vi "NI 9263 DOUBLE TASK.vi"(8 "error in":errorcluster, 10 "MODULE NAME 2":string="CDR_AO2", 11 "MODULE NAME":string="CDR_AO1") -> (0 "error out":errorcluster, 3 "task out":refnum<k21>)   [LabVIEW 2019]
uses:
  <vilib>/DAQmx/create/channels.llb/DAQmx Create Channel (AO-Voltage-Basic).vi
  <resource>/objmgr/daqmx.rc
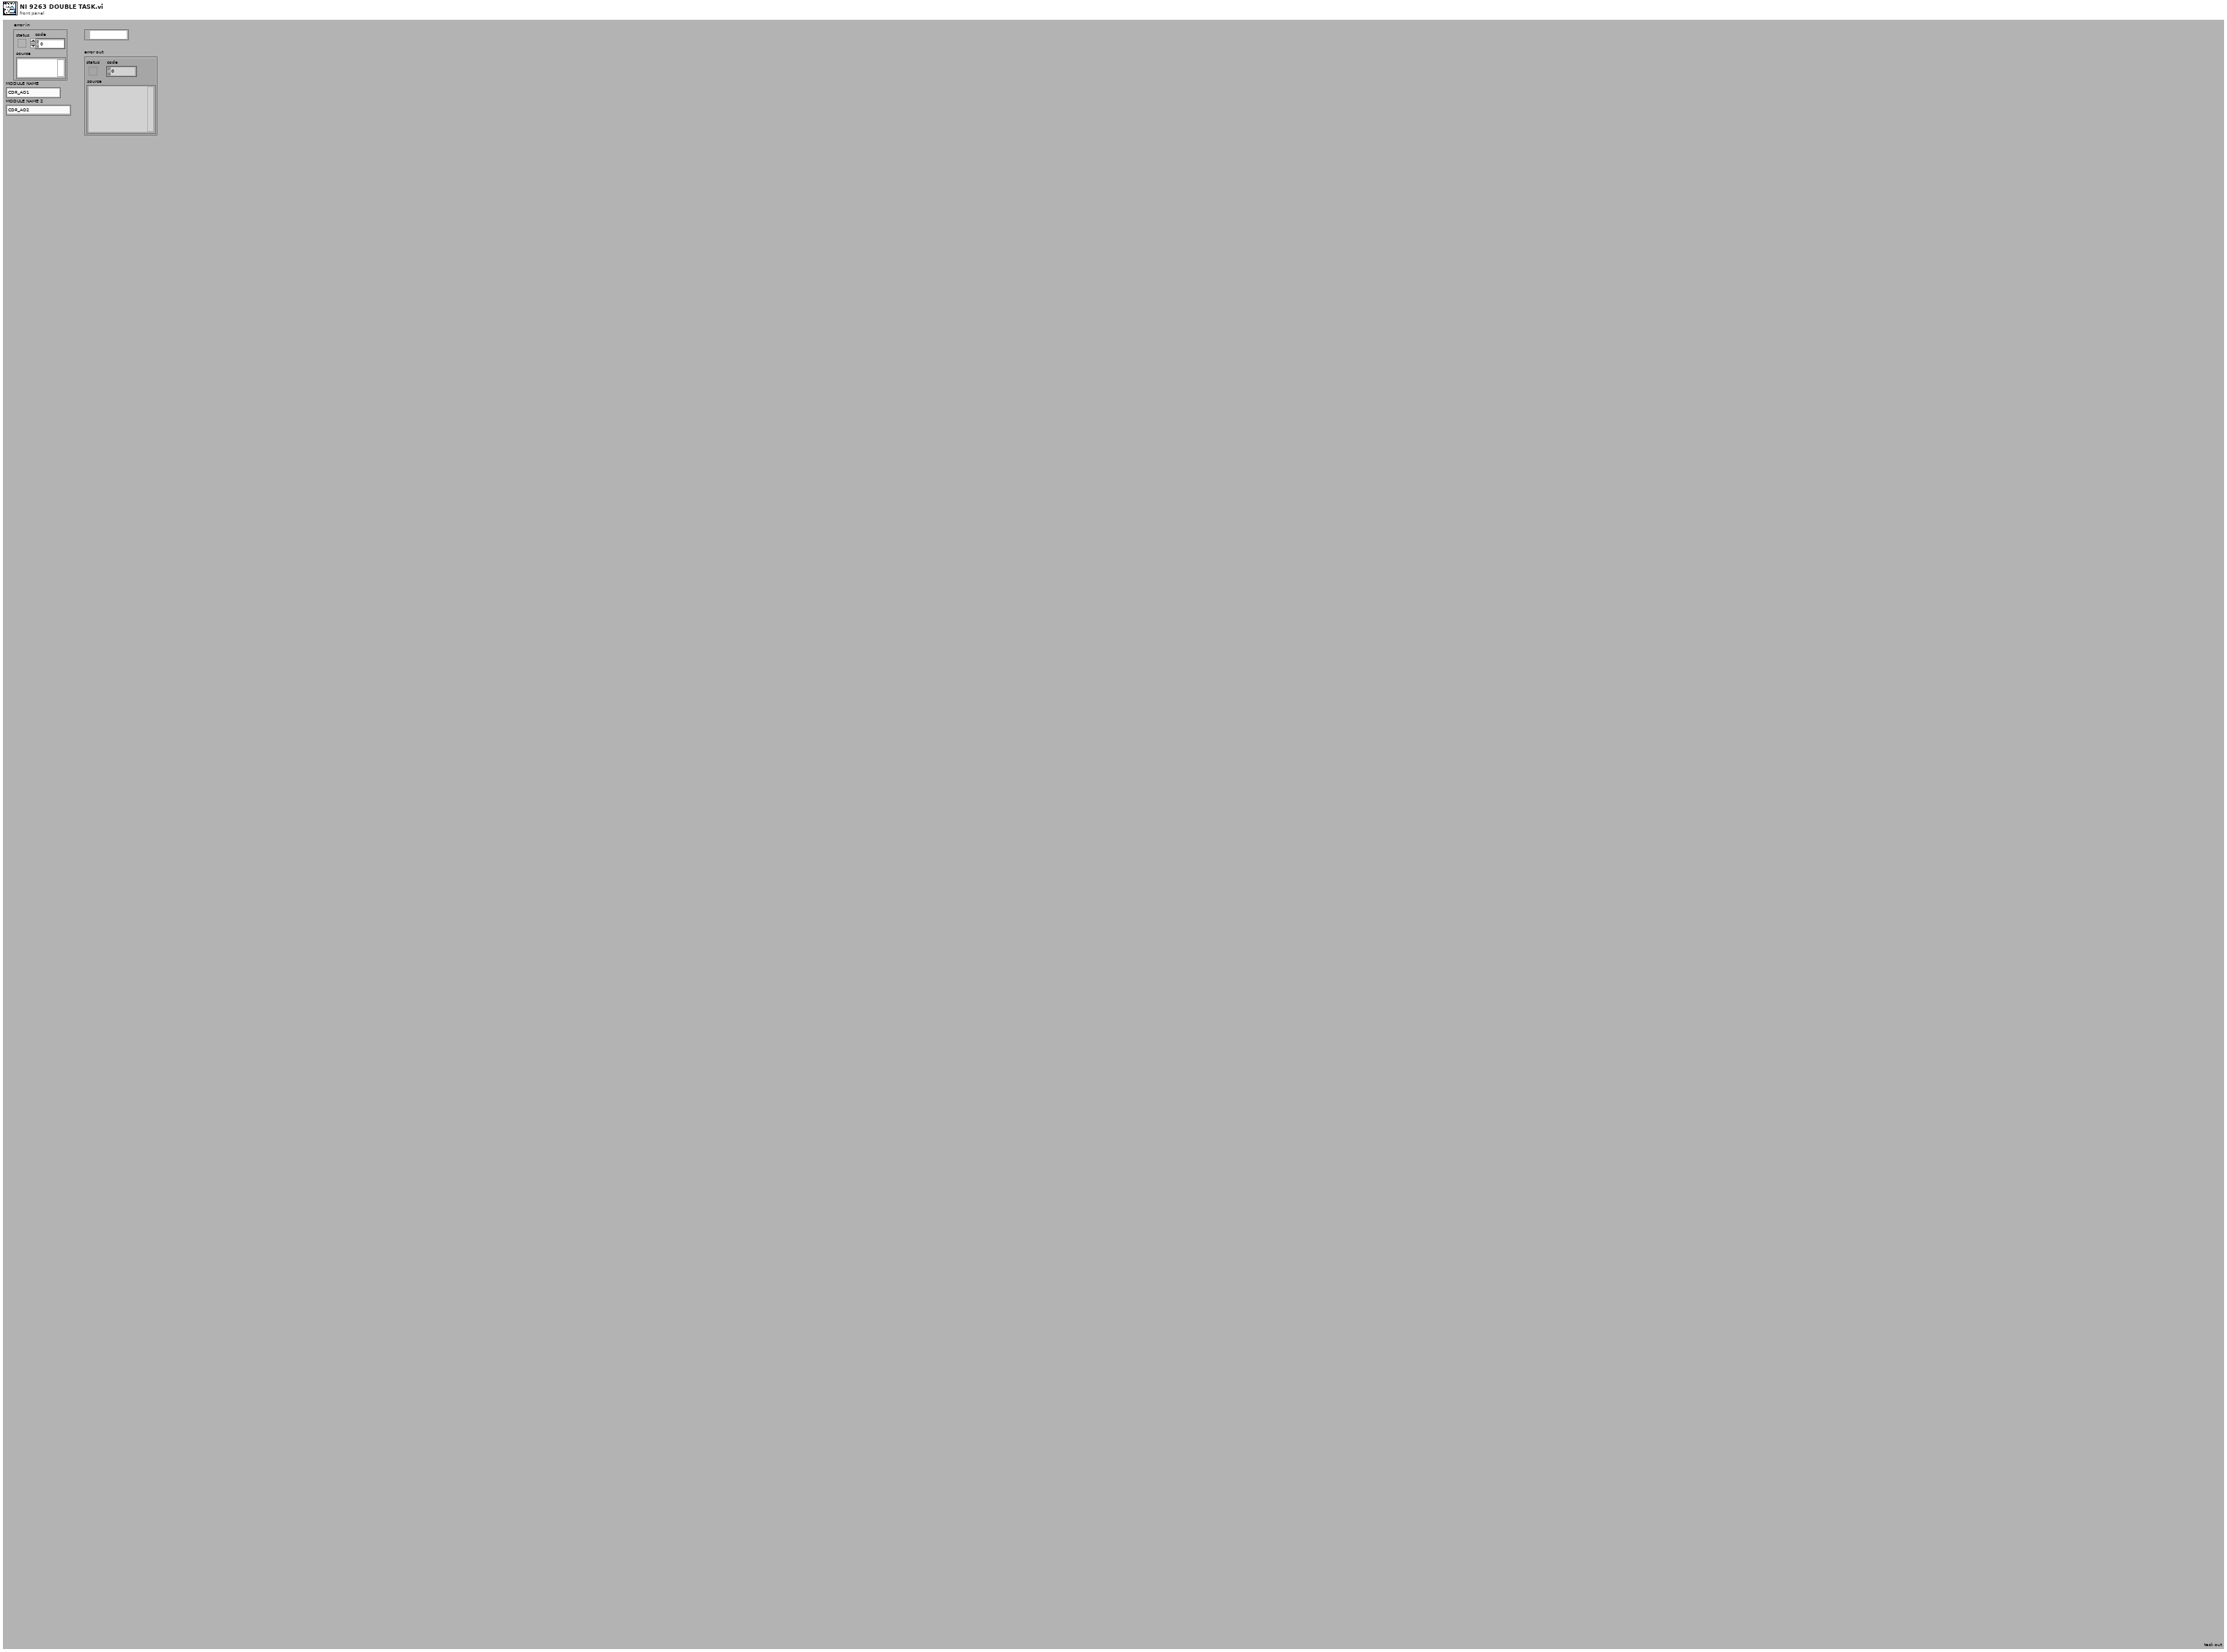
[diagram p1: front panel]
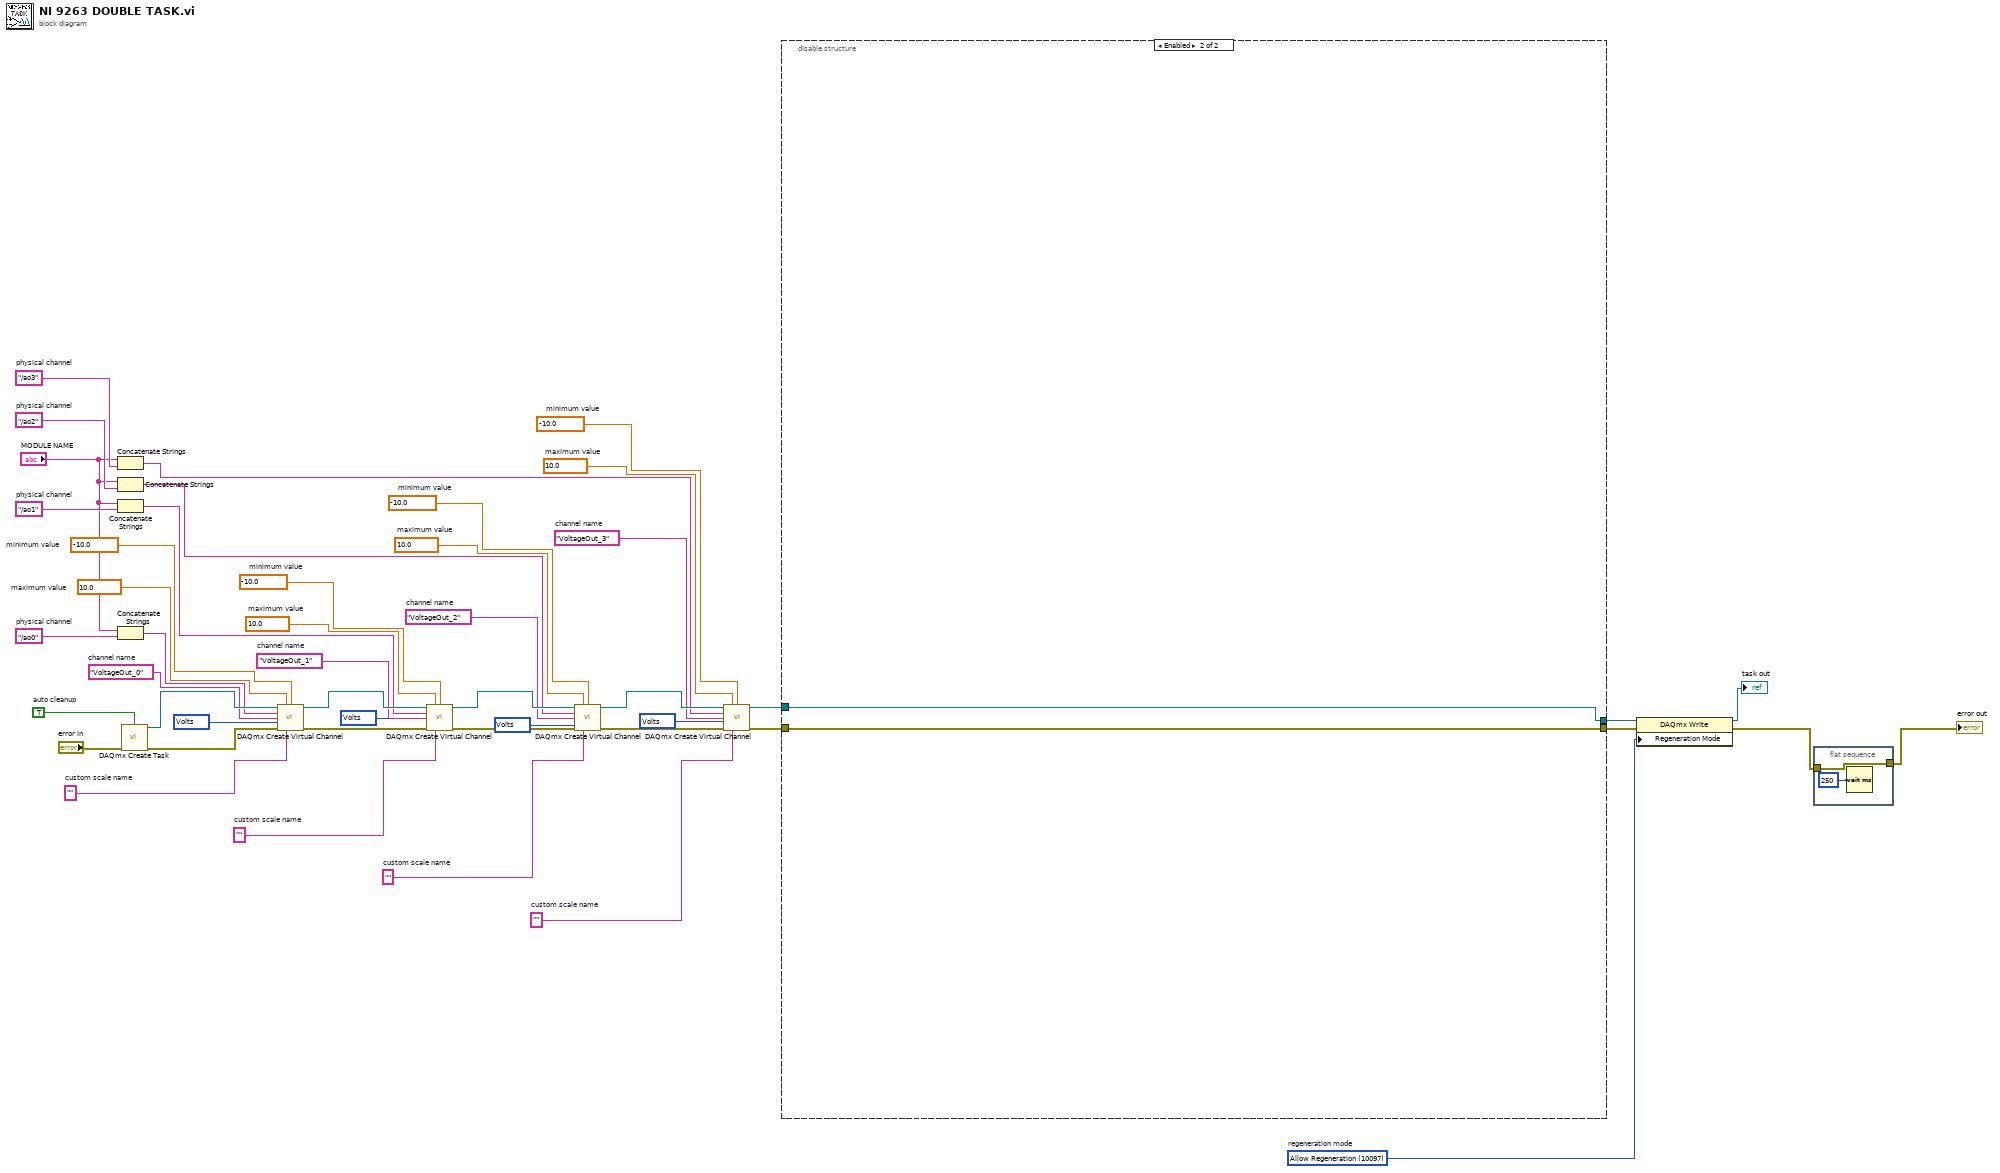
[diagram p0: block diagram]
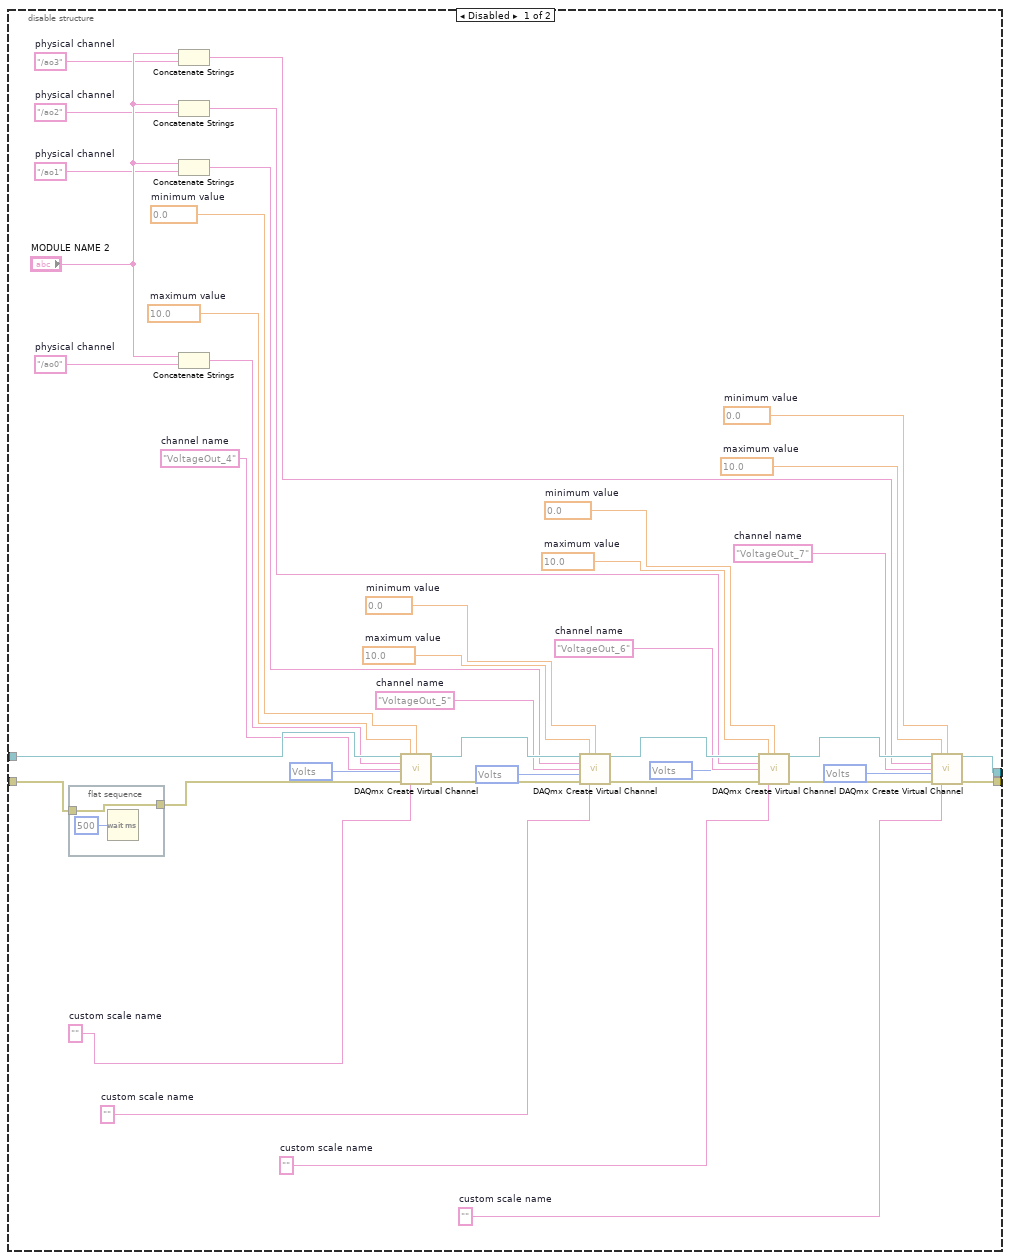
[diagram p2: hidden frame]
diagram:
  w1 = 10348 items=["Volts"=10348, "From Custom Scale"=10065] ("units")
  w2 = 10348 items=["Volts"=10348, "From Custom Scale"=10065] ("units")
  w3 = 10348 items=["Volts"=10348, "From Custom Scale"=10065] ("units")
  w4 = 10348 items=["Volts"=10348, "From Custom Scale"=10065] ("units")
  w21 = 10097 items=["Allow Regeneration"=10097, "Do Not Allow Regeneration"=10158]  # regeneration mode
  w23 = "VoltageOut_3"  # channel name
  w24 = ""  # custom scale name
  w25 = -10.0  # minimum value
  w26 = 10.0  # maximum value
  w12 = "/ao3"  # physical channel
  w28 = "VoltageOut_2"  # channel name
  w30 = ""  # custom scale name
  w31 = -10.0  # minimum value
  w32 = 10.0  # maximum value
  w14 = "/ao2"  # physical channel
  w34 = "VoltageOut_1"  # channel name
  w36 = ""  # custom scale name
  w37 = -10.0  # minimum value
  w38 = 10.0  # maximum value
  w15 = "/ao1"  # physical channel
  w40 = "VoltageOut_0"  # channel name
  w42 = ""  # custom scale name
  w43 = -10.0  # minimum value
  w44 = 10.0  # maximum value
  w17 = "/ao0"  # physical channel
  w46 = TRUE  # auto cleanup
  n1 = Concatenate Strings("MODULE NAME", w12) -> (w11:string)
  n2 = Concatenate Strings("MODULE NAME", w14) -> (w13:string)
  n3 = Concatenate Strings("MODULE NAME", w15) -> (w10:string)
  n4 = Concatenate Strings("MODULE NAME", w17) -> (w16:string)
  n5 = call <vilib>:"DAQmx Create Task.vi"("auto cleanup"=w46, "error in"="error in") -> ("task out"=w45:refnum<k21>, "error out"=w47:errorcluster)  [unwired: 12 in]
  n6 = call-poly <vilib>:"DAQmx Create Virtual Channel.vi"("task in"=w45, "maximum value"=w44, "minimum value"=w43, "physical channels"=w16, "name to assign"=w40, "units"=w4, "error in"=w47, "custom scale name"=w42) -> ("task out"=w39:refnum<k21>, "error out"=w41:errorcluster)  [unwired: 6 in]
  n7 = call-poly <vilib>:"DAQmx Create Virtual Channel.vi"("task in"=w39, "maximum value"=w38, "minimum value"=w37, "physical channels"=w10, "name to assign"=w34, "units"=w3, "error in"=w41, "custom scale name"=w36) -> ("task out"=w33:refnum<k21>, "error out"=w35:errorcluster)  [unwired: 6 in]
  n8 = call-poly <vilib>:"DAQmx Create Virtual Channel.vi"("task in"=w33, "maximum value"=w32, "minimum value"=w31, "physical channels"=w13, "name to assign"=w28, "units"=w2, "error in"=w35, "custom scale name"=w30) -> ("task out"=w27:refnum<k21>, "error out"=w29:errorcluster)  [unwired: 6 in]
  n9 = call-poly <vilib>:"DAQmx Create Virtual Channel.vi"("task in"=w27, "maximum value"=w26, "minimum value"=w25, "physical channels"=w11, "name to assign"=w23, "units"=w1, "error in"=w29, "custom scale name"=w24) -> ("task out"=w22:refnum<k21>, "error out"=w5:errorcluster)  [unwired: 6 in]
  n10 = disable-structure shown="Enabled" {
    disable-tunnel: w22 -> [w87 w91]
    disable-tunnel: [w83 w91] -> w19
    disable-tunnel: [w82 w90] -> w18
    disable-tunnel: w5 -> [w54 w90]
    frame Disabled {
      w48 = ""  # custom scale name
      w49 = 10348 items=["Volts"=10348, "From Custom Scale"=10065] ("units")
      w50 = 10348 items=["Volts"=10348, "From Custom Scale"=10065] ("units")
      w51 = 10348 items=["Volts"=10348, "From Custom Scale"=10065] ("units")
      w52 = 10348 items=["Volts"=10348, "From Custom Scale"=10065] ("units")
      w64 = "VoltageOut_7"  # channel name
      w65 = 0.0  # minimum value
      w66 = 10.0  # maximum value
      w56 = "/ao3"  # physical channel
      w68 = "VoltageOut_6"  # channel name
      w70 = 0.0  # minimum value
      w71 = 10.0  # maximum value
      w58 = "/ao2"  # physical channel
      w73 = "VoltageOut_5"  # channel name
      w75 = 0.0  # minimum value
      w76 = 10.0  # maximum value
      w60 = "/ao1"  # physical channel
      w78 = "VoltageOut_4"  # channel name
      w80 = 0.0  # minimum value
      w81 = 10.0  # maximum value
      w62 = "/ao0"  # physical channel
      w84 = ""  # custom scale name
      w85 = ""  # custom scale name
      w86 = ""  # custom scale name
      n11 = flat-sequence {
        tunnel: [w88] -> w53
        tunnel: w54 -> [w88]
        frame #0 {
          n12 = Wait (ms)(milliseconds to wait=u32 500) -> ()  [unwired: 1 out]
        }
      }
      n13 = Concatenate Strings("MODULE NAME 2", w56) -> (w55:string)
      n14 = Concatenate Strings("MODULE NAME 2", w58) -> (w57:string)
      n15 = Concatenate Strings("MODULE NAME 2", w60) -> (w59:string)
      n16 = Concatenate Strings("MODULE NAME 2", w62) -> (w61:string)
      n17 = call-poly <vilib>:"DAQmx Create Virtual Channel.vi"("task in"=w87, "maximum value"=w81, "minimum value"=w80, "physical channels"=w61, "name to assign"=w78, "units"=w52, "error in"=w53, "custom scale name"=w48) -> ("task out"=w77:refnum<k21>, "error out"=w79:errorcluster)  [unwired: 6 in]
      n18 = call-poly <vilib>:"DAQmx Create Virtual Channel.vi"("task in"=w77, "maximum value"=w76, "minimum value"=w75, "physical channels"=w59, "name to assign"=w73, "units"=w51, "error in"=w79, "custom scale name"=w86) -> ("task out"=w72:refnum<k21>, "error out"=w74:errorcluster)  [unwired: 6 in]
      n19 = call-poly <vilib>:"DAQmx Create Virtual Channel.vi"("task in"=w72, "maximum value"=w71, "minimum value"=w70, "physical channels"=w57, "name to assign"=w68, "units"=w50, "error in"=w74, "custom scale name"=w85) -> ("task out"=w67:refnum<k21>, "error out"=w69:errorcluster)  [unwired: 6 in]
      n20 = call-poly <vilib>:"DAQmx Create Virtual Channel.vi"("task in"=w67, "maximum value"=w66, "minimum value"=w65, "physical channels"=w55, "name to assign"=w64, "units"=w49, "error in"=w69, "custom scale name"=w84) -> ("task out"=w83:refnum<k21>, "error out"=w82:errorcluster)  [unwired: 6 in]
    }
    frame Enabled {
    }
  }
  n21 = property class="DAQmx Write"(reference=w19, error in=w18, "Regeneration Mode"=w21) -> (reference out=→"task out":refnum<k21>, error out=w7:errorcluster)
  n22 = flat-sequence {
    tunnel: [w92] -> w6
    tunnel: w7 -> [w92]
    frame #0 {
      n23 = Wait (ms)(milliseconds to wait=u32 250) -> ()  [unwired: 1 out]
    }
  }
  "error out" <- w6
